vi "Get Data.vi"(8 "error in":errorcluster, 11 "CRDS in":refnum<class "CRDS.lvclass">) -> (0 "error out":errorcluster, 3 "CRDS out":refnum<class "CRDS.lvclass">)   [LabVIEW 2015, in "CRDS Lib.lvlib" / "CRDS.lvclass"]
doc: "The base CRD <b>Get Data</b> implementation only handles the coadding of traces. If the property <b>Coadd</b> == 1, then this VI will do nothing."
uses:
  CRDS.lvclass
  CRDS.lvclass/CRDS.ctl
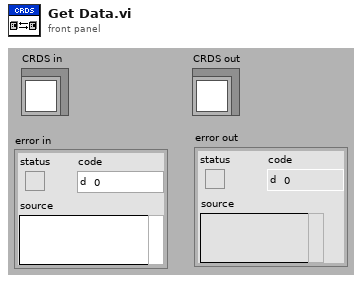
[diagram p1: front panel]
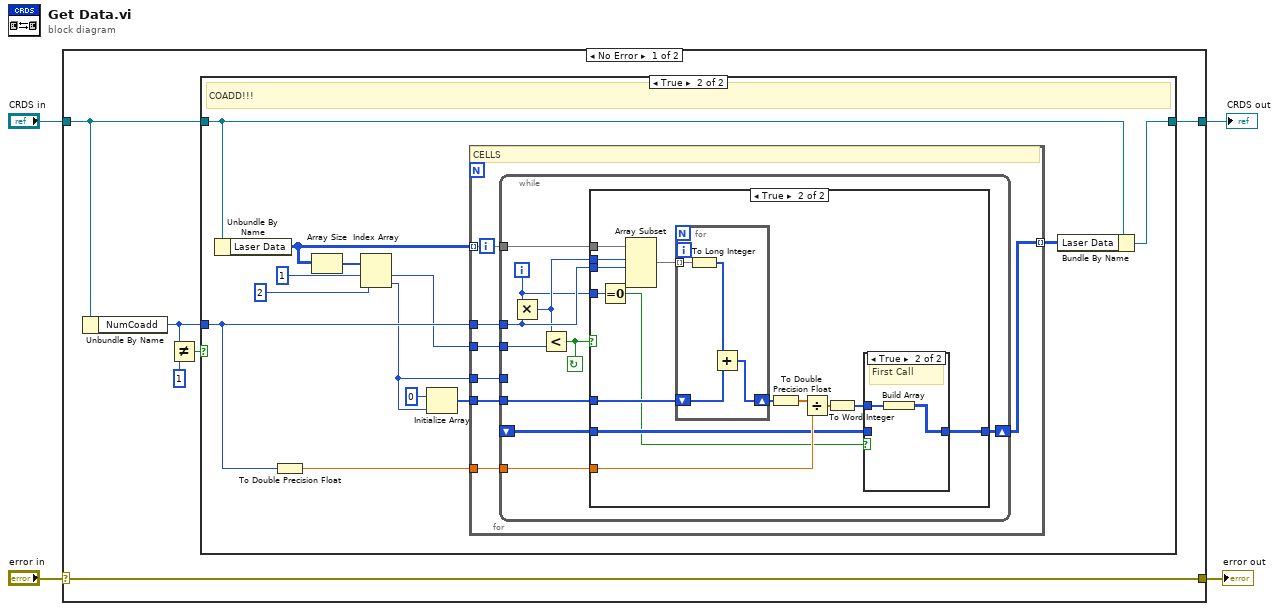
[diagram p0: block diagram]
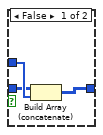
[diagram p4: hidden frame]
diagram:
  n1 = case shown="No Error" "error in" {
    selector: "error in" -> [w10 w66]
    tunnel: [w5 w67] -> w3
    tunnel: "CRDS in" -> [w6 w67]
    tunnel: [w10 w66] -> w2
    frame No Error {
      n2 = Unbundle By Name(w6) -> ("NumCoadd"=w7:i32)
      n3 = Not Equal?(x=w7, y=1) -> (x != y?=w8:bool)
      n4 = case shown="True" w8 {
        tunnel: w7 -> [_ w18]
        tunnel: w6 -> [w11 w24]
        tunnel: [w11 w23] -> w5
        frame False {
          # "NO COADDING"
        }
        frame True {
          # "COADD!!!"
          n5 = Unbundle By Name(w24) -> ("Laser Data"=w22:i16[][][])
          n6 = To Double Precision Float(number=w18) -> (double precision float=w17:dbl)
          n7 = Array Size(array=w22) -> (size(s)=w21:i32[])
          n8 = Index Array(array=w21, index #1=1 ("index"), index #2=2 ("index")) -> (element #1=w15:i32, element #2=w14:i32)
          n9 = Initialize Array(0 ("element"), w14) -> (w19:i32[])
          n10 = for {
            tunnel: w22 -> [w31] mode=indexing
            tunnel: w18 -> [w30]
            tunnel: w14 -> [w29]
            tunnel: w19 -> [w28]
            tunnel: w17 -> [w27]
            tunnel: w15 -> [w26]
            tunnel: [w25] -> w16 mode=indexing
            # "CELLS"
            n11 = while {
              tunnel: w31 -> [w41]
              tunnel: w30 -> [w40]
              tunnel: w29 -> [_]
              tunnel: w28 -> [w39]
              tunnel: w27 -> [w38]
              tunnel: w26 -> [w36]
              shift-right: [w34] -> w25
              shift-left: _ -> [w33]
              i -> [w32]
              stop <- w35 continue-if-true
              n12 = Multiply(x=w32, y=w40) -> (x*y=w37:i32)
              n13 = Less?(x=w37, y=w36) -> (x < y?=w35:bool)
              n14 = case shown="True" w35 {
                tunnel: w41 -> [_ w56]
                tunnel: w40 -> [_ w55]
                tunnel: w39 -> [_ w53]
                tunnel: w38 -> [_ w50]
                tunnel: w37 -> [_ w48]
                tunnel: [w42 w46] -> w34
                tunnel: w33 -> [w42 w45]
                tunnel: w32 -> [_ w44]
                frame False {
                  # "LAST CALL"
                }
                frame True {
                  n15 = Equal To 0?(x=w44) -> (x = 0?=w43:bool)
                  n16 = Array Subset(array=w56, index (row)=w48, length (row)=w55) -> (w54:i16[][])  [unwired: 2 in]
                  n17 = for {
                    tunnel: w54 -> [w63] mode=indexing
                    shift-right: [w64] -> w52
                    shift-left: w53 -> [w65]
                    n18 = To Long Integer(number=w63) -> (32bit integer=w62:i32[])
                    n19 = Add(x=w62, y=w65) -> (x+y=w64:i32[])
                  }
                  n20 = To Double Precision Float(number=w52) -> (double precision float=w51:dbl[])
                  n21 = Divide(x=w51, y=w50) -> (x/y=w49:dbl[])
                  n22 = To Word Integer(number=w49) -> (16bit integer=w47:i16[])
                  n23 = case shown="True" w43 {
                    tunnel: w47 -> [w59 w61]
                    tunnel: [w58 w60] -> w46
                    tunnel: w45 -> [w57 _]
                    frame False {
                      n24 = Build Array (concatenate)(w57, w59) -> (w58:i16[][])
                    }
                    frame True {
                      # "First Call"
                      n25 = Build Array(w61) -> (w60:i16[][])
                    }
                  }
                }
              }
            }
          }
          n26 = Bundle By Name(cluster=w24, "Laser Data"=w16) -> (w23:refnum<class "CRDS.lvclass">)
        }
      }
    }
    frame Error {
    }
  }
  "error out" <- w2
  "CRDS out" <- w3
